vi "1sec-for.vi"() -> ()   [LabVIEW 2009]
panel:
  out "Numeric":i32
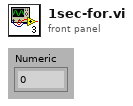
[diagram p1: front panel]
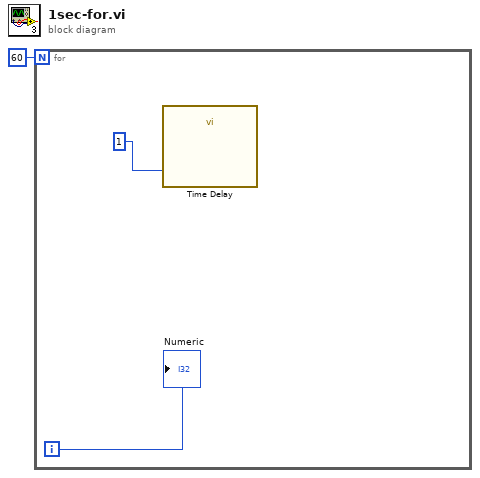
[diagram p0: block diagram]
diagram:
  n1 = for {
    N: 60 -> [_]
    i -> [w2]
    n2 = call "Time Delay"("Delay Time (s)"=1) -> ()  [unwired: 10 in, 1 out]
    "Numeric" <- w2
  }
